vi "_20_Sample_qsns_06[36].vi"() -> ()   [LabVIEW 2020]
panel:
  out "Numeric 4":u8
  in  "Numeric 3":u8
  in  "Numeric 2":u8
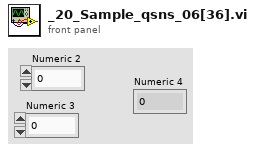
[diagram p1: front panel]
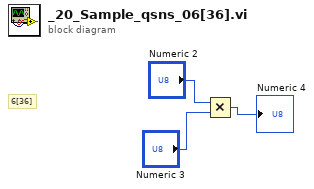
[diagram p0: block diagram]
diagram:
  # "6[36]"
  n1 = Multiply(x="Numeric 2", y="Numeric 3") -> (x*y=→"Numeric 4":u8)
